vi "Get Active Instrument.vi"(8 "error in (no error)":errorcluster, 9 "Instrument Index":i32, 10 "Category Index":i32, 11 "StoreUI in":refnum<class "StoreUI.lvclass">) -> (0 "error out":errorcluster, 2 "Item":refnum<class "Generic Item.lvclass">, 3 "StoreUI out":refnum<class "StoreUI.lvclass">)   [LabVIEW 2015, in "StoreUI.lvlib" / "StoreUI.lvclass"]
uses:
  StoreUI.lvclass
  Classes/Generic Item/Generic Item.lvclass
  StoreUI.lvclass/StoreUI.ctl
  VI Store/VIStore Actor/VIStore.lvclass/VIStore.ctl
  Classes/Category/Category.lvclass
  VI Store/VIStore Actor/VIStore.lvclass
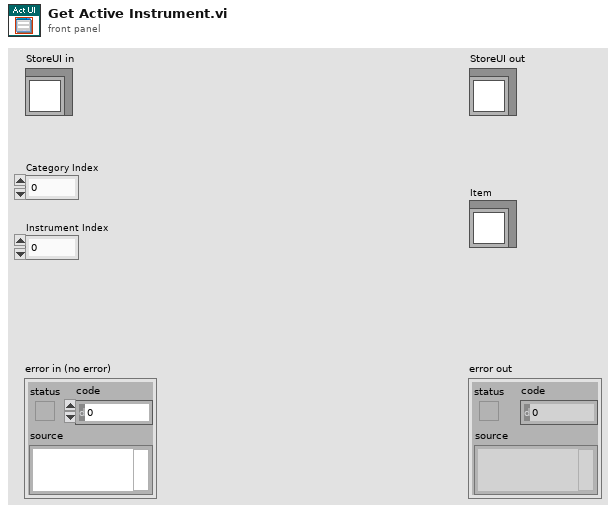
[diagram p1: front panel]
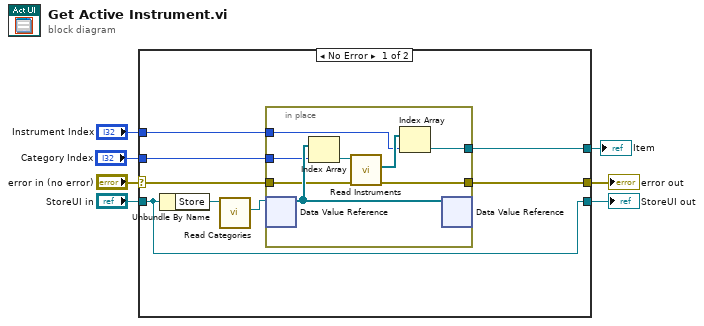
[diagram p0: block diagram]
diagram:
  n1 = case shown="No Error" "error in (no error)" {
    selector: "error in (no error)" -> [w12 w25]
    tunnel: [w11 w25] -> w6
    tunnel: [w15 w24] -> w4
    tunnel: "StoreUI in" -> [w15 w24]
    tunnel: "Category Index" -> [w14 _]
    tunnel: "Instrument Index" -> [w13 _]
    tunnel: [w10 _] -> w1
    frame No Error {
      n2 = Unbundle By Name(w15) -> ("Store"=w9:refnum<class "VIStore.lvclass">)
      n3 = call "Read Categories.vi"("VIStore in"=w9) -> ("Categories"=w8:refnum<data-value>)  [unwired: 8 in, 2 out]
      n4 = in-place {
        in-place-border: w14 -> [w20]
        in-place-border: w13 -> [w19]
        in-place-border: w12 -> [w18]
        in-place-border: [w17] -> w11
        in-place-border: [w16] -> w10
        n5 = in-place-dvr #1(w8) -> (w22:refnum<class "Category.lvclass">[])  [unwired: 1 out]
        n6 = Index Array(array=w22, index=w20) -> (element=w23:refnum<class "Category.lvclass">)
        n7 = call-dynamic "Read Instruments.vi"("error in (no error)"=w18, "Category in"=w23) -> ("error out"=w17:errorcluster, "Instruments"=w21:refnum<class "Generic Item.lvclass">[])  [unwired: 7 in, 1 out]
        n8 = Index Array(array=w21, index=w19) -> (element=w16:refnum<class "Generic Item.lvclass">)
        n9 = in-place-dvr #1(w22) -> ()  [unwired: 2 out]
      }
    }
    frame Error {
    }
  }
  "error out" <- w6
  "StoreUI out" <- w4
  "Item" <- w1
